vi "BLE_Sample - Test2.vi"() -> ()   [LabVIEW 2020]
uses:
  C:/Users/Kevin/Desktop/BLE/BLELib.dll
  BLELib.dll
panel:
  out "device list":T1(array[cluster])
  out "Array 2":string[](array[string])
  out "Array":string[](array[string])
  out "StartDeviceWatcher":string
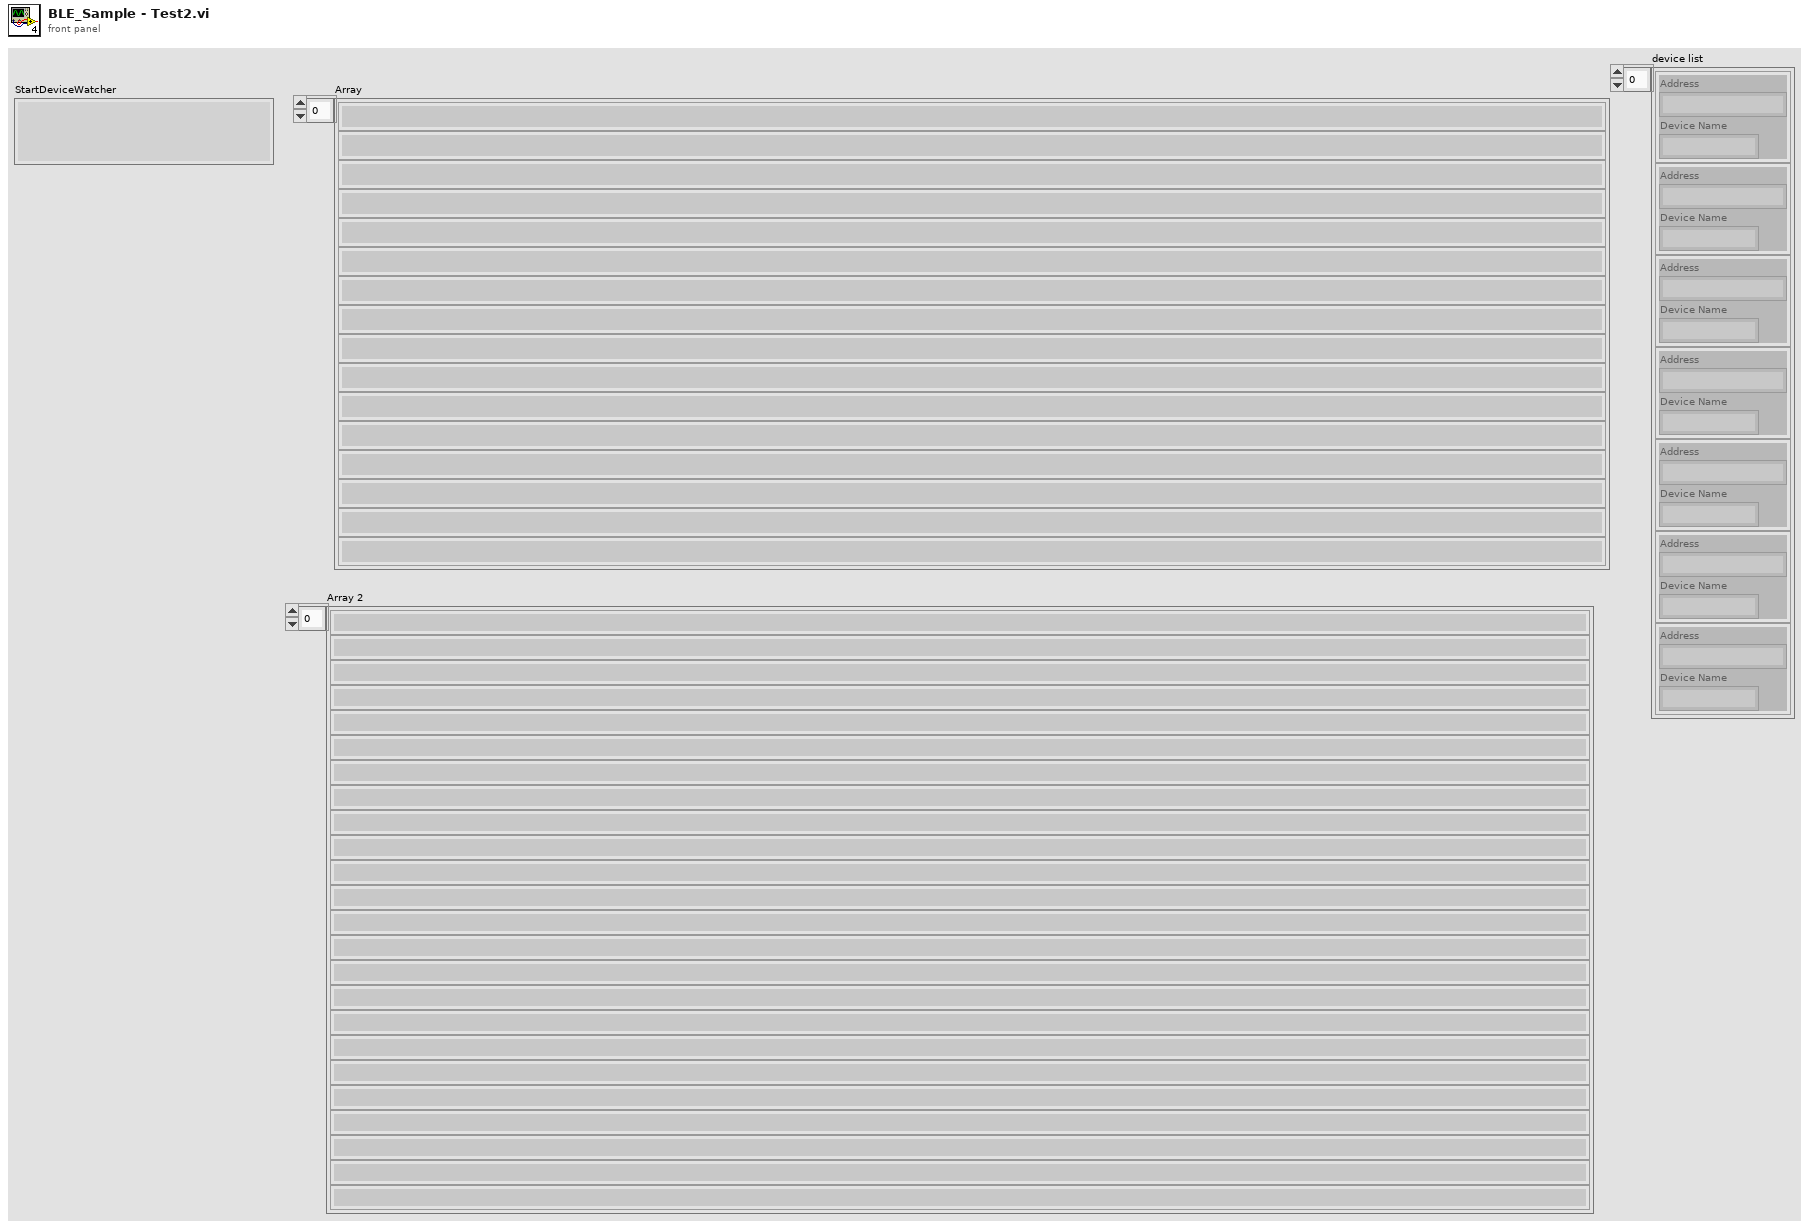
[diagram p1: front panel]
types:
  T1 = cluster{"Address":string, "Device Name":string}[]
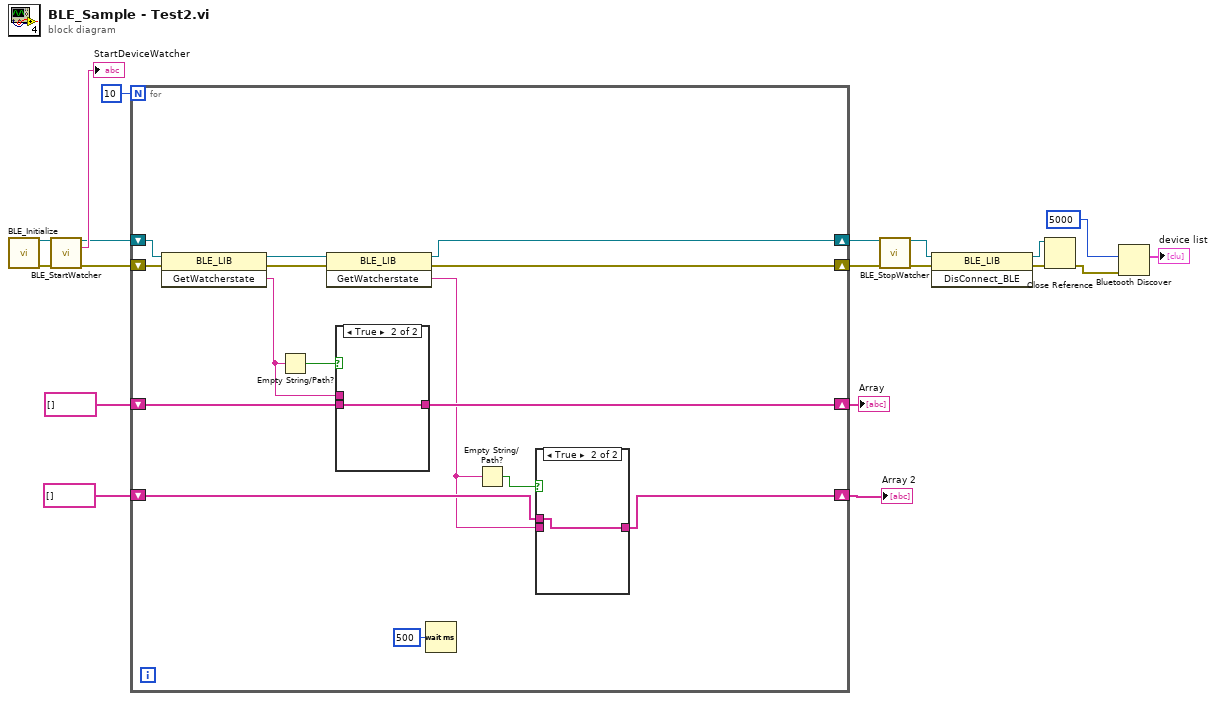
[diagram p0: block diagram]
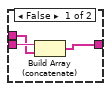
[diagram p2: hidden frame]
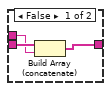
[diagram p3: hidden frame]
diagram:
  n1 = call "BLE_Initialize.vi"() -> (".NET Refnum out"=w19:refnum<k24>, "error out"=w18:errorcluster)  [unwired: 14 in]
  n2 = call "BLE_StartWatcher.vi"(".NET Refnum in"=w19, "error in (no error)"=w18) -> (".NET Refnum out"=w14:refnum<k24>, "StartDeviceWatcher"=→"StartDeviceWatcher":string, "error out"=w13:errorcluster)  [unwired: 11 in]
  n3 = for {
    N: 10 -> [_]
    shift-right: [w28] -> w12
    shift-left: w14 -> [w32]
    shift-right: [w29] -> w11
    shift-left: w13 -> [w33]
    shift-right: [w25] -> w6
    shift-left: string[] [] -> [w26]
    shift-right: [w20] -> w4
    shift-left: string[] [] -> [w22]
    n4 = invoke class="BLE_LIB" method="GetWatcherstate"(reference=w32, error in=w33) -> (reference out=w30:refnum<k24>, error out=w31:errorcluster, "GetWatcherstate"=w24:string)  [unwired: 1 in]
    n5 = Empty String/Path?(string/path=w24) -> (empty?=w27:bool)
    n6 = invoke class="BLE_LIB" method="GetWatcherstate"(reference=w30, error in=w31) -> (reference out=w28:refnum<k24>, error out=w29:errorcluster, "GetWatcherstate"=w21:string)  [unwired: 1 in]
    n7 = case shown="True" w27 {
      tunnel: w26 -> [w41 w42]
      tunnel: [w40 w42] -> w25
      tunnel: w24 -> [w39 _]
      frame False {
        n8 = Build Array (concatenate)(w41, w39) -> (w40:string[])
      }
      frame True {
      }
    }
    n9 = Wait (ms)(milliseconds to wait=u32 500) -> ()  [unwired: 1 out]
    n10 = Empty String/Path?(string/path=w21) -> (empty?=w23:bool)
    n11 = case shown="True" w23 {
      tunnel: w21 -> [w37 _]
      tunnel: [w36 w38] -> w20
      tunnel: w22 -> [w35 w38]
      frame False {
        n12 = Build Array (concatenate)(w37, w35) -> (w36:string[])
      }
      frame True {
      }
    }
  }
  "Array" <- w6
  "Array 2" <- w4
  n13 = call "BLE_StopWatcher.vi"(".NET Refnum in"=w12, "error in (no error)"=w11) -> (".NET Refnum out"=w9:refnum<k24>, "error out"=w10:errorcluster)  [unwired: 11 in, 1 out]
  n14 = invoke class="BLE_LIB" method="DisConnect_BLE"(reference=w9, error in=w10) -> (reference out=w16:refnum<k24>, error out=w17:errorcluster)  [unwired: 1 in, 1 out]
  n15 = Close Reference(reference=w16, error in (no error)=w17) -> (error out=w3:errorcluster)
  n16 = Bluetooth Discover(8:w3, 10:5000 ("time limit ms (10000)")) -> (2:→"device list":T1)  [unwired: 2 out]
